vi "Update Wilt GUI.vi"(0 "Dryer In":T1 {"Night Cycle Count" format="%04d"; "Dryer Details"."Stop Dryer" items=["NO", "YES"]; "Dryer Details"."24 Hour Water Injection" items=["NO", "YES"]; "Dryer Details"."Run w/o Newfi" items=["NO", "YES"]; "Day Cycle Count" format="%04d"}, 1 "Day Shift?":bool, 2 "Enum":T5, 3 "Station Index":i32=13, 5 "Station Label In":string, 7 "New Dryer Details In":T2 {"Stop Dryer" items=["NO", "YES"]; "24 Hour Water Injection" items=["NO", "YES"]; "Run w/o Newfi" items=["NO", "YES"]}, 9 "Com Port In":u8=13, 11 "Dryer Status Serial Data In":T3, 12 "Agilent Data In":dbl[](array[numeric])=[1.0, 2.0, 3.0, 4.0, 5.0], 13 "Audit Alert":bool) -> (4 "Dryer Out 2":T1 {"Night Cycle Count" format="%04d"; "Dryer Details"."Stop Dryer" items=["NO", "YES"]; "Dryer Details"."24 Hour Water Injection" items=["NO", "YES"]; "Dryer Details"."Run w/o Newfi" items=["NO", "YES"]; "Day Cycle Count" format="%04d"}, 8 "New Dryer Testing File Init":bool, 10 "Restart Ready?":bool)   [LabVIEW 2012]
uses:
  Update Wilt GUI Control.ctl
  Dryer.ctl
  Dryer Details.ctl
  Dryer Com Port Info.ctl
  Dryer Status Ctrl.ctl
  Globals Wilt.vi
panel:
  in  "Tab Control":enum32{"Out", "In"}(tab)
  out "Dryer Breakout":T1 {"Night Cycle Count" format="%04d"; "Dryer Details"."Stop Dryer" items=["NO", "YES"]; "Dryer Details"."24 Hour Water Injection" items=["NO", "YES"]; "Dryer Details"."Run w/o Newfi" items=["NO", "YES"]; "Day Cycle Count" format="%04d"}
  in  "Dryer Out":T1 {"Night Cycle Count" format="%04d"; "Dryer Details"."Stop Dryer" items=["NO", "YES"]; "Dryer Details"."24 Hour Water Injection" items=["NO", "YES"]; "Dryer Details"."Run w/o Newfi" items=["NO", "YES"]; "Day Cycle Count" format="%04d"}
  out "Dryer Out.Sample Record(t, CC, Tc, ASCII, Status, L1,L2,Trmb,V{,V2,SW} )":string[](array[string])
  out "Dryer Out.Sample Record(t, CC, Tc, ASCII, Status, L1,L2,Trmb,V{,V2,SW} ) 2":string[](array[string])
  out "Dryer Breakout":T1 {"Night Cycle Count" format="%04d"; "Dryer Details"."Stop Dryer" items=["NO", "YES"]; "Dryer Details"."24 Hour Water Injection" items=["NO", "YES"]; "Dryer Details"."Run w/o Newfi" items=["NO", "YES"]; "Day Cycle Count" format="%04d"}
  in  "Dryer":T1 {"Night Cycle Count" format="%04d"; "Dryer Details"."Stop Dryer" items=["NO", "YES"]; "Dryer Details"."24 Hour Water Injection" items=["NO", "YES"]; "Dryer Details"."Run w/o Newfi" items=["NO", "YES"]; "Day Cycle Count" format="%04d"}
  # "D"
  # "N"
  # "D"
  # "N"
  # "D"
  # "N"
  # "D"
  # "N"
  # "D"
  # "N"
  # "D"
  # "N"
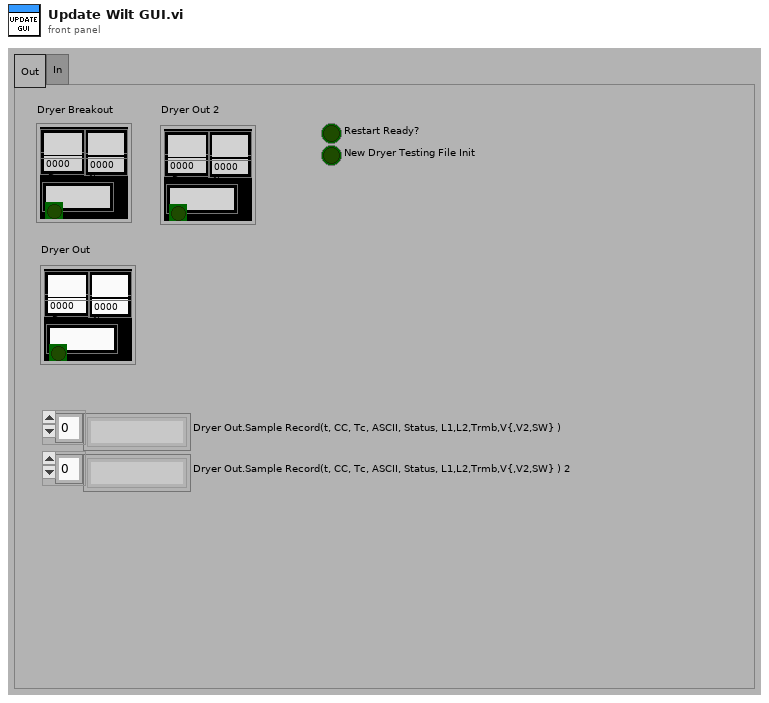
[diagram p1: front panel]
types:
  T1 = typedef "Dryer.ctl" = cluster{"Lab ID":string, "Day Cycle Count":i32, "Station Label":string, "Dryer Details":T2, "Sample Record ":string[], "Hist Record ":string[][], "Status Color":u32, "Boolean":bool, "Com Port":u8, "Bad Com Count":i32, "Current Run Start Time":dbl, "Night Cycle Count":i32, "Station Index":i32, "Cycle Index":string, "Audit Alert":bool}
  T2 = typedef "Dryer Details.ctl" = cluster{"Station":string, "Cycle Count Day":string, "Status":string, "Debug ASCII":string, "Notes":string, "Lab ID":string, "Total Time On":string, "TR Number":string, "Cycle Count Night":string, "Time On Day":string, "Time On Night":string, "Run w/o Newfi":i32, "24 Hour Water Injection":i32, "Stop Dryer":i32}
  T3 = typedef "Dryer Com Port Info.ctl" = cluster{"Color":u32, "Last Read Status":T4, "Command:Data":string, "Com Port":u8, "Time(S)":dbl, "Err Count":u32}
  T4 = typedef "Dryer Status Ctrl.ctl" = enum16{"Cycle Not Started", "Cycle Running", "Paused", "Cycle Completed", "Eval Mode Entered", "Err", "Pause (No GEA2)"}
  T5 = typedef "Update Wilt GUI Control.ctl" = enum16{"Init Station Number", "Update Detail Data", "Update Status", "Init Com Port Num", "Update Sample Info", "Reset All Cycles"}
  T6 = cluster{"New Dryer Details In":T2, "Station Label In":string, "Com Port In":u8, "Agilent Data In":dbl[], "Dryer Status Serial Data In":T3, "Restart Ready?":bool, "Dryer Out":T1, "Temperature Fault":bool, "Station Index":i32, "Audit Alert":bool, "Day Shift?":bool}
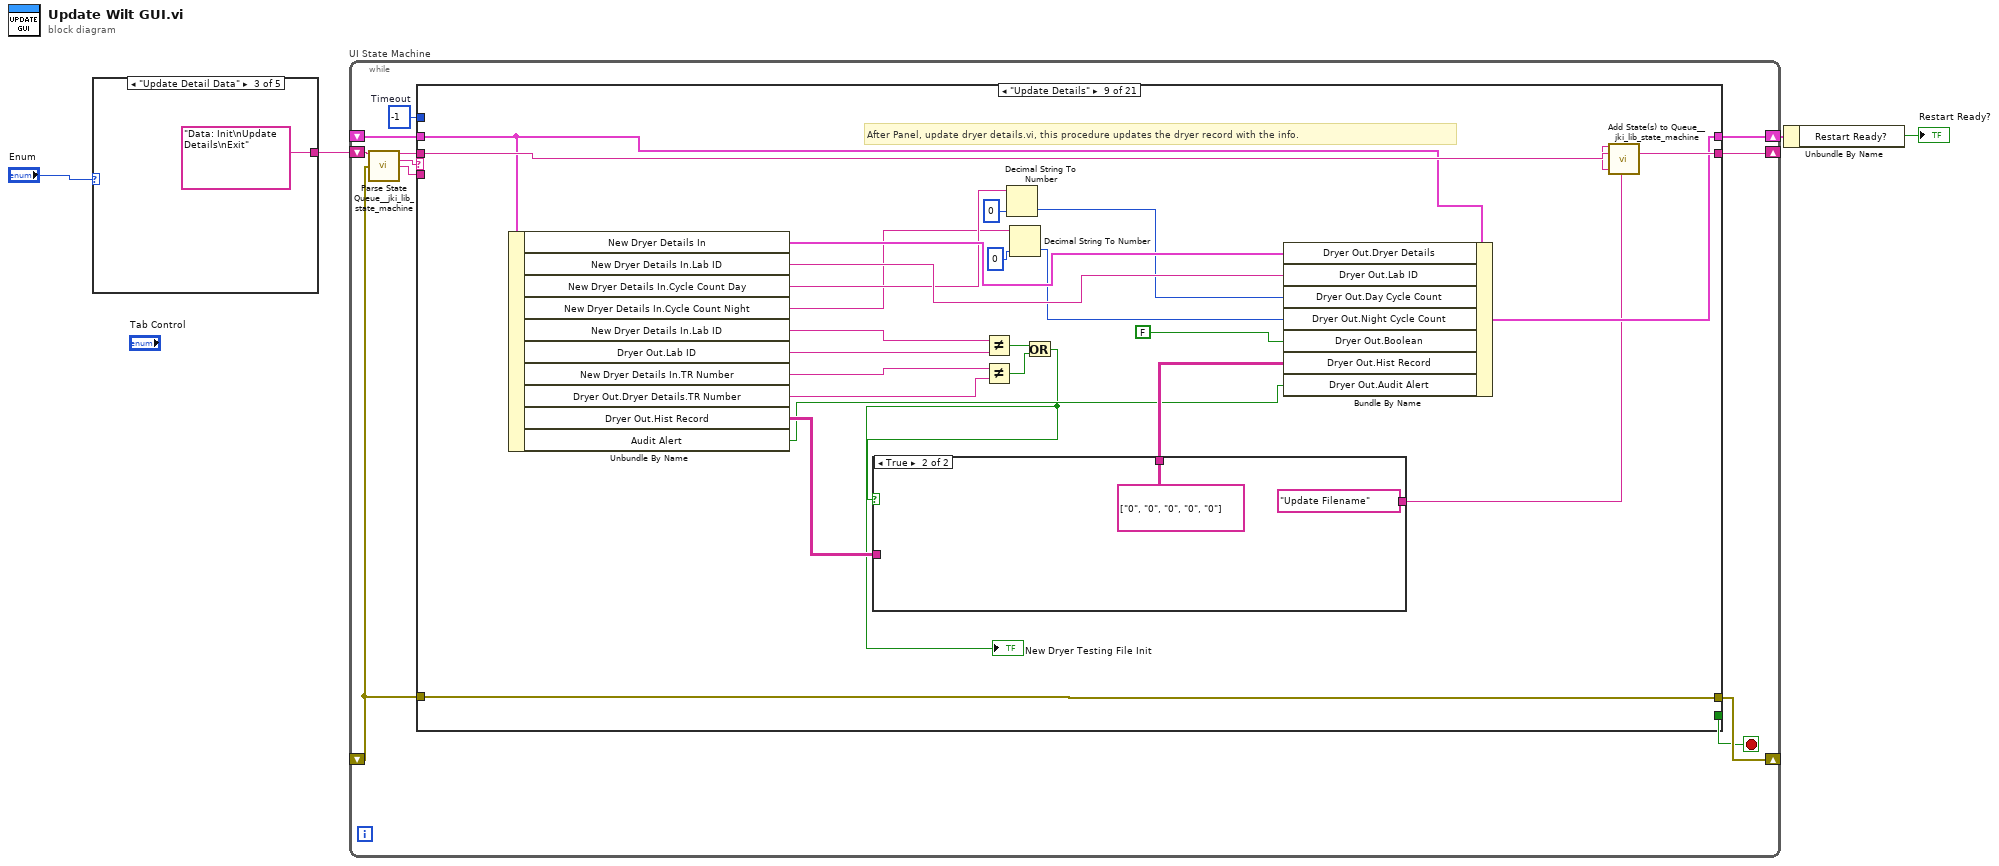
[diagram p0: block diagram]
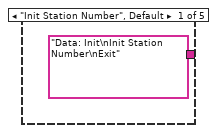
[diagram p2: hidden frame]
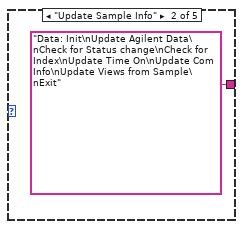
[diagram p3: hidden frame]
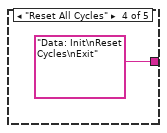
[diagram p4: hidden frame]
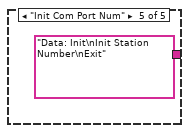
[diagram p5: hidden frame]
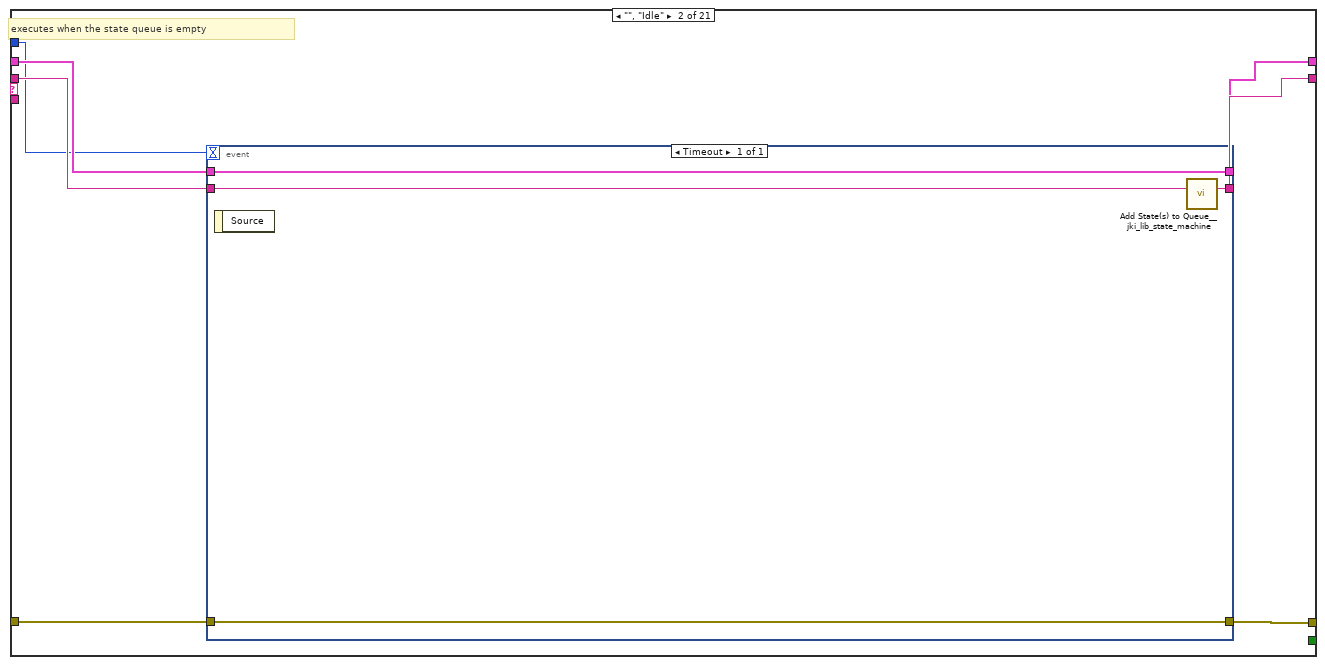
[diagram p7: hidden frame]
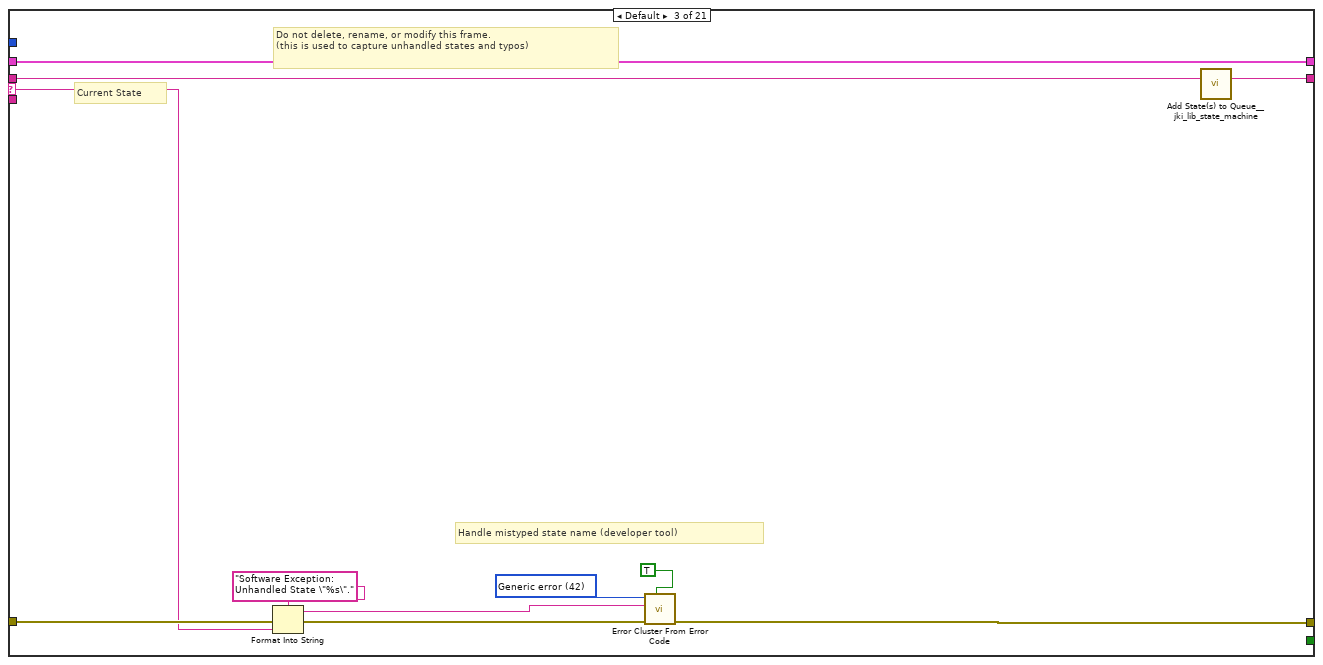
[diagram p8: hidden frame]
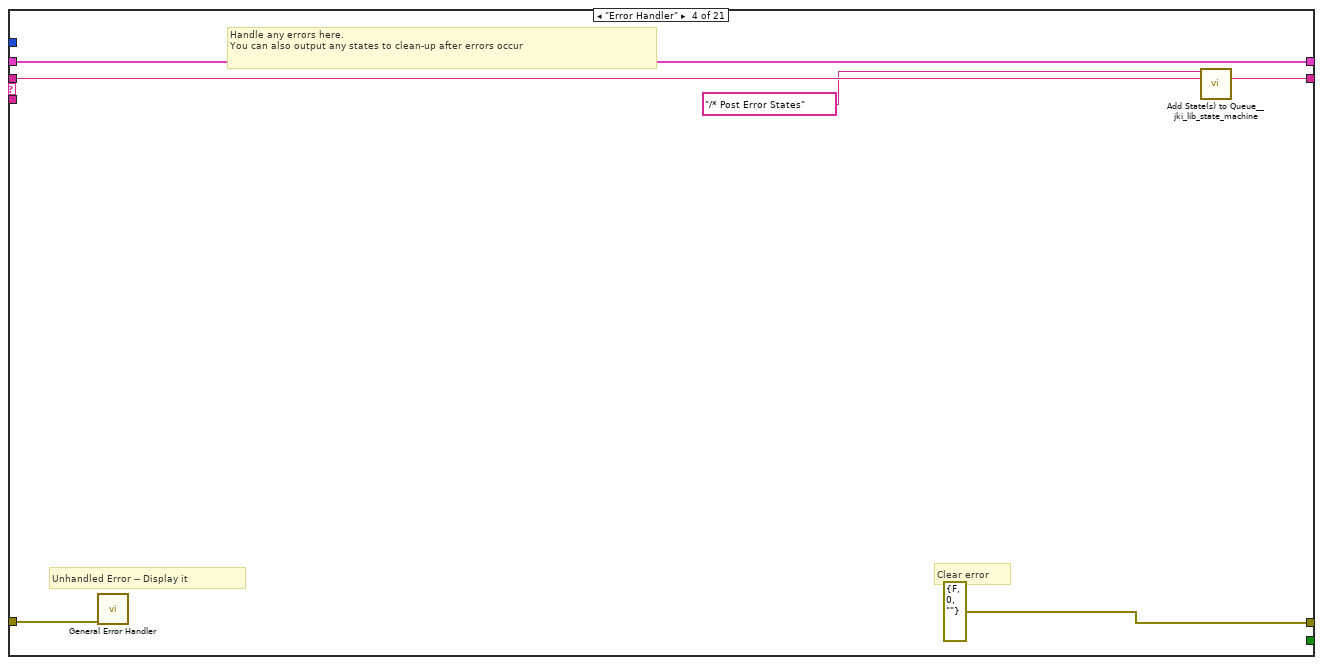
[diagram p9: hidden frame]
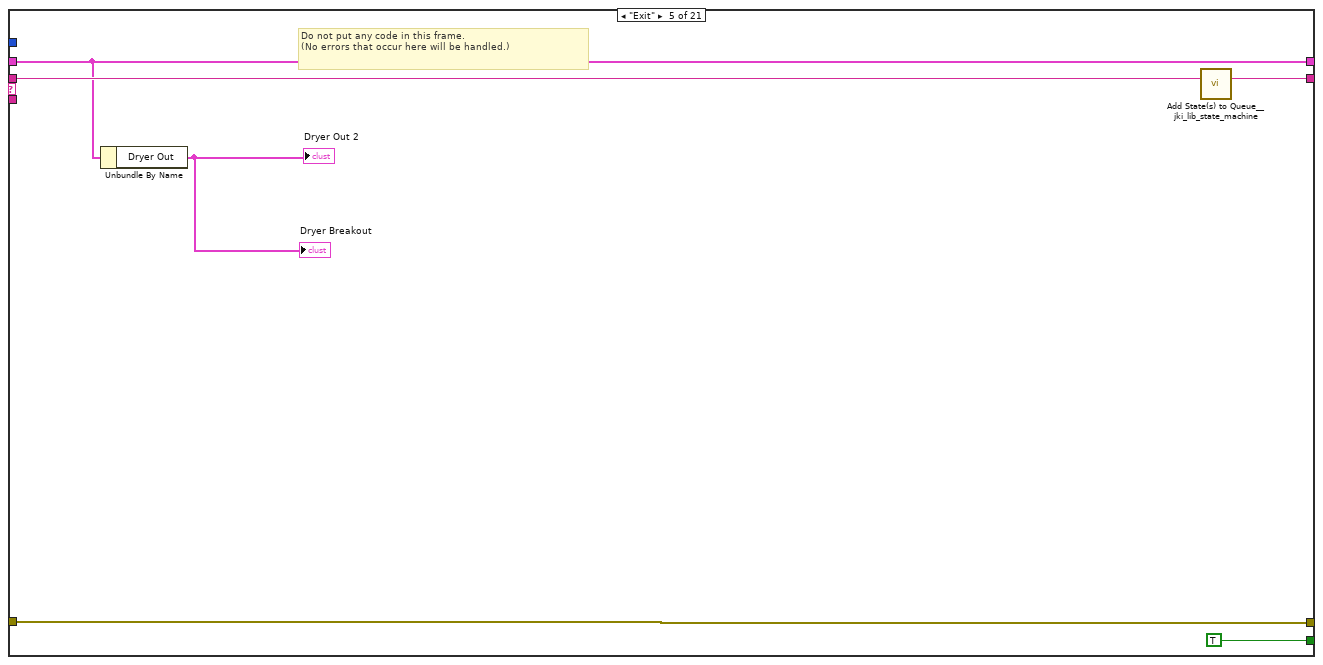
[diagram p10: hidden frame]
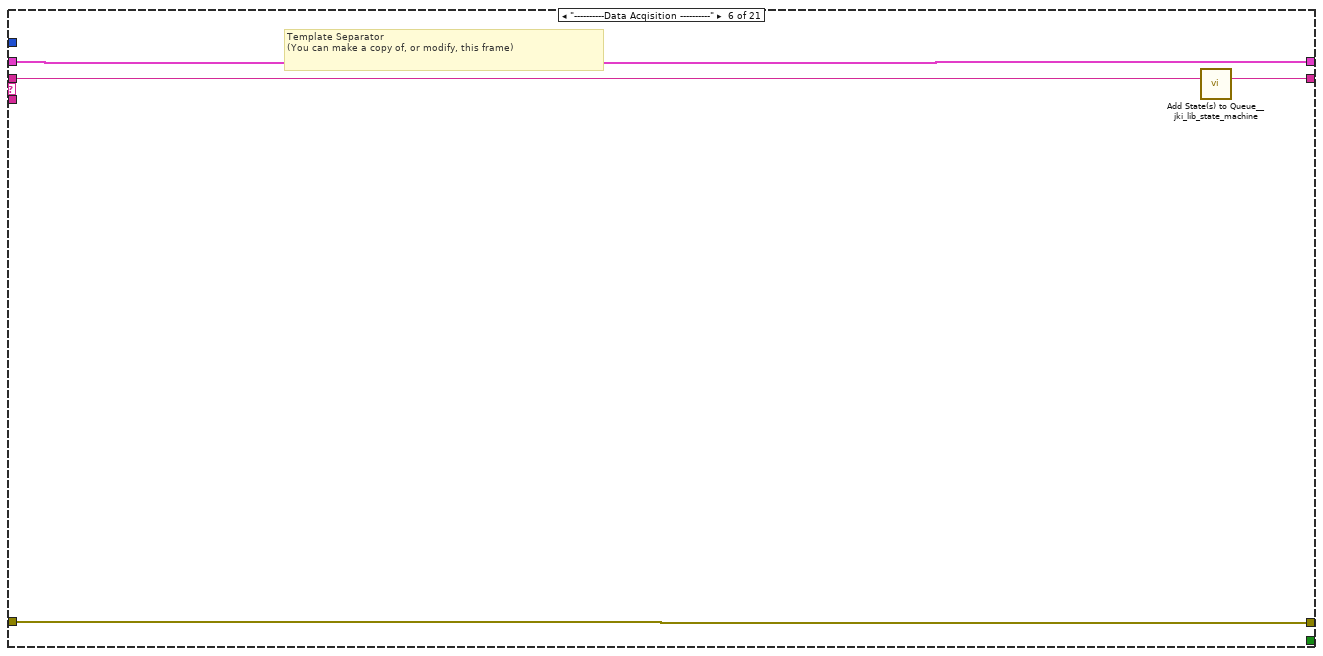
[diagram p11: hidden frame]
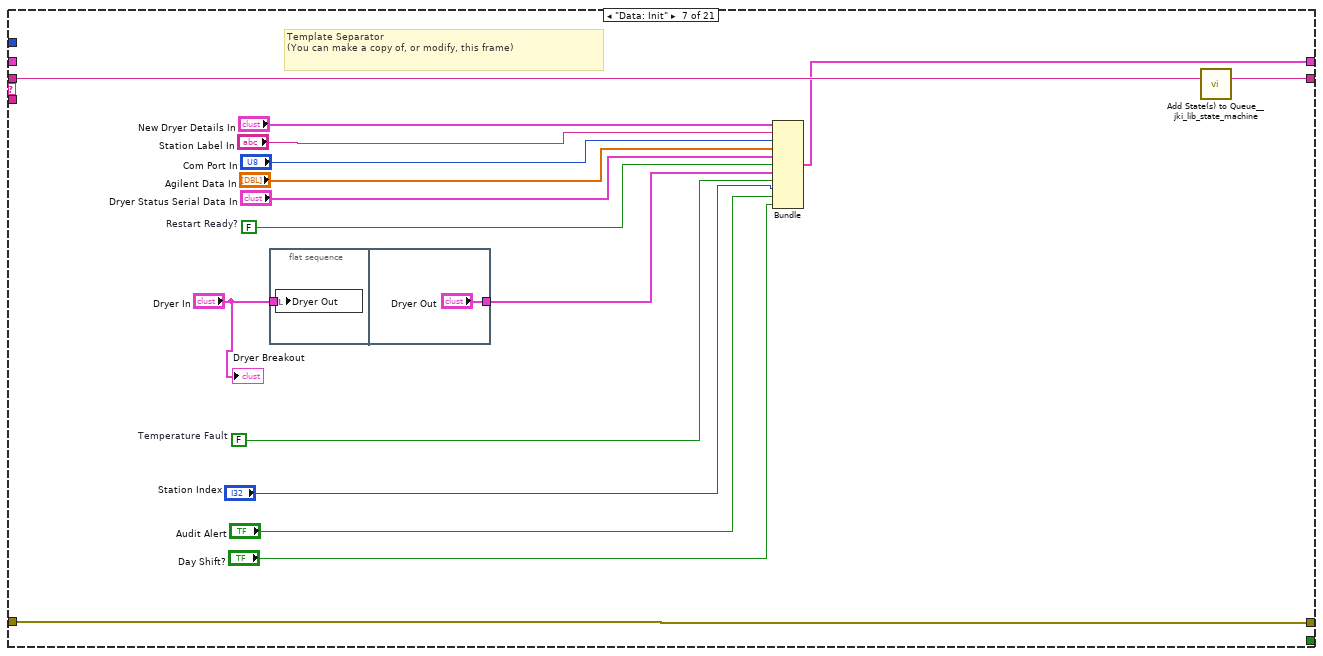
[diagram p12: hidden frame]
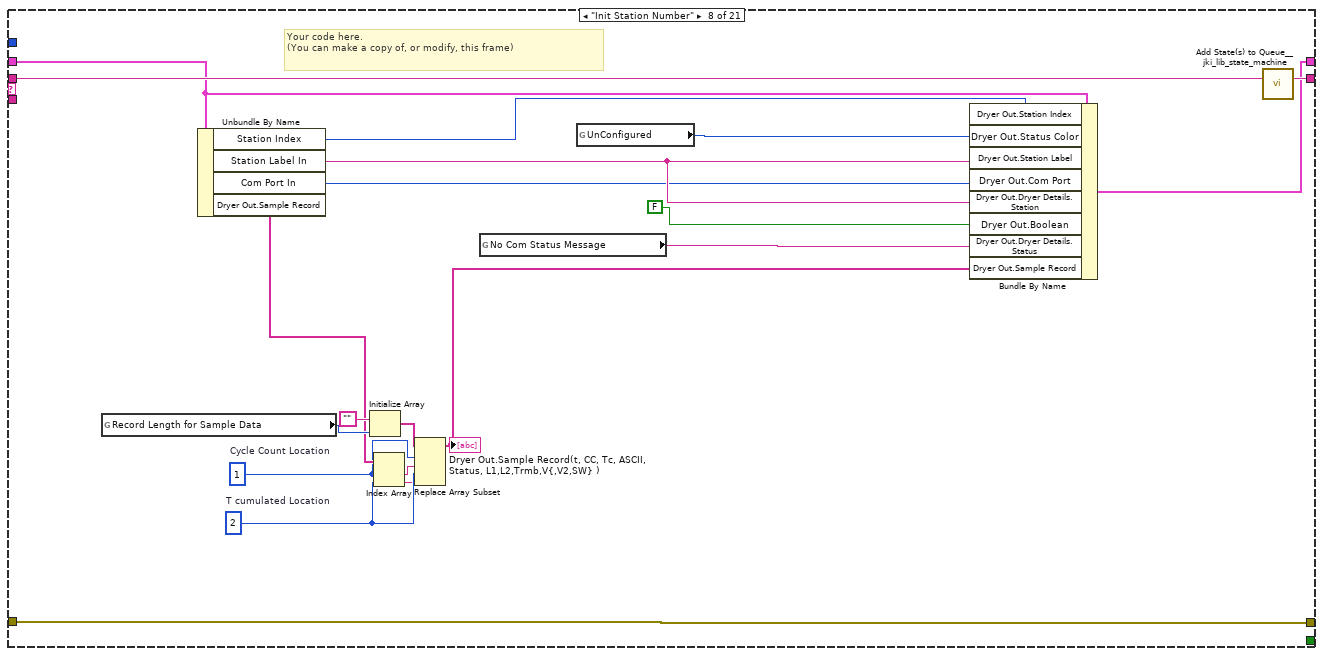
[diagram p13: hidden frame]
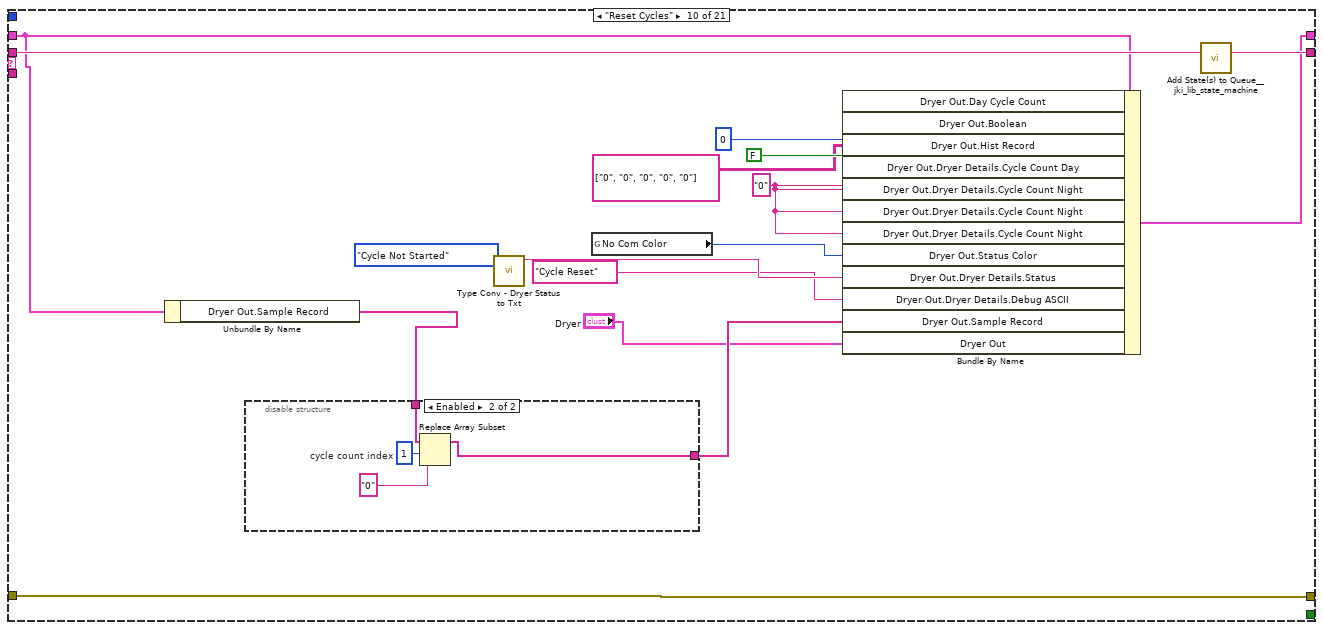
[diagram p15: hidden frame]
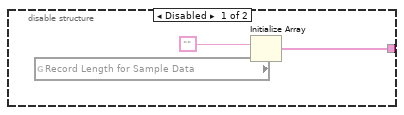
[diagram p16: hidden frame]
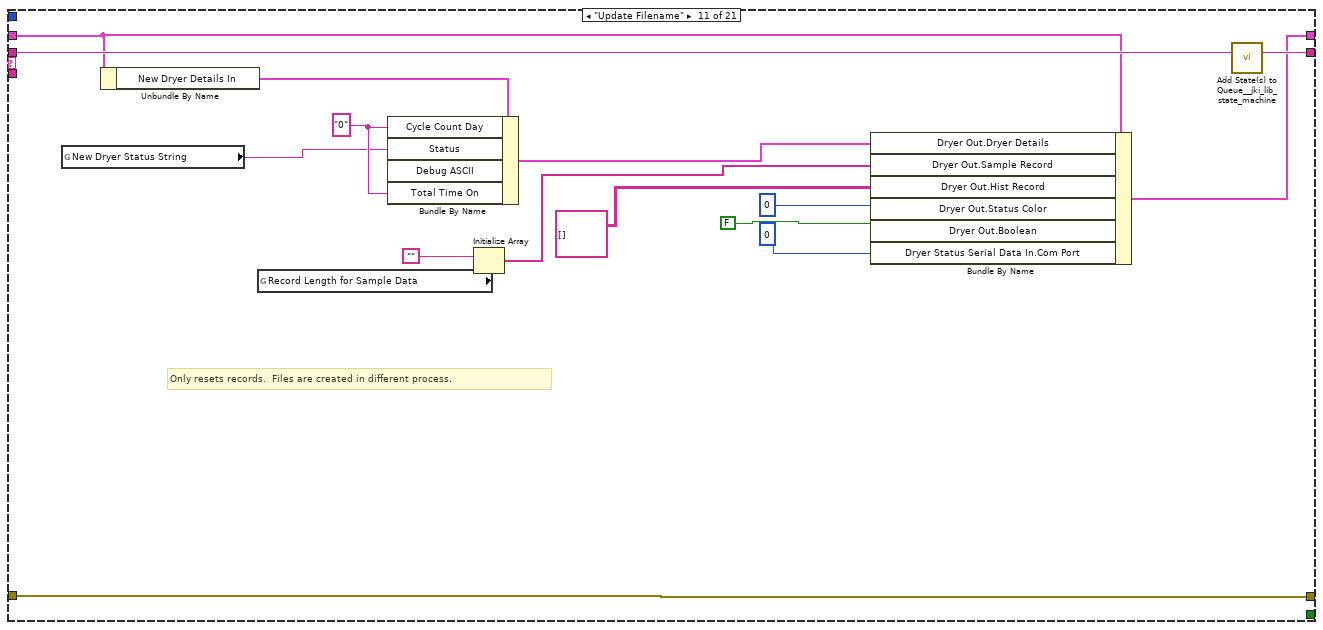
[diagram p17: hidden frame]
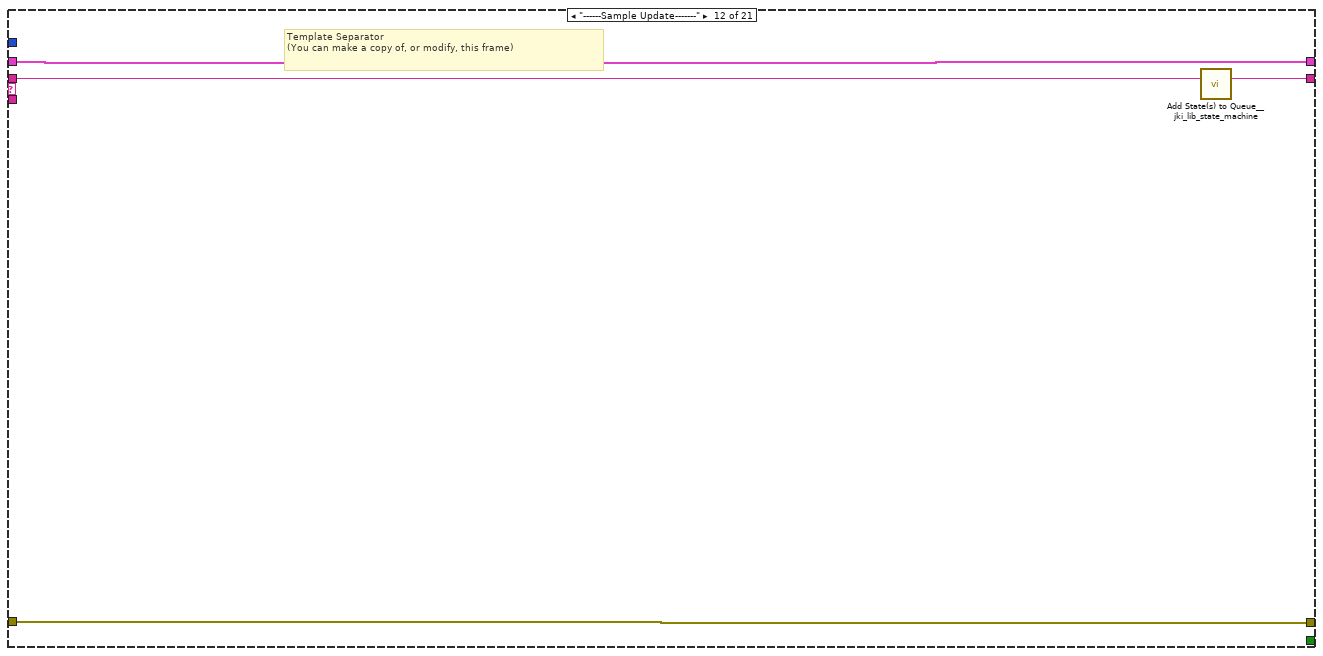
[diagram p18: hidden frame]
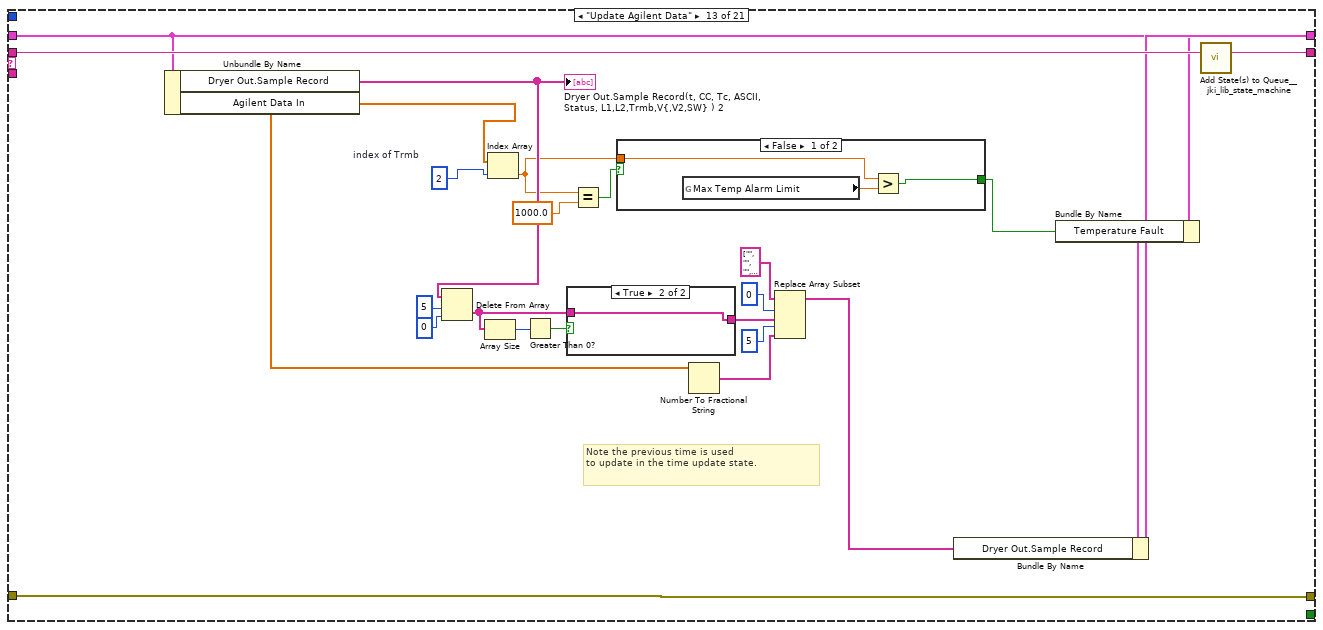
[diagram p19: hidden frame]
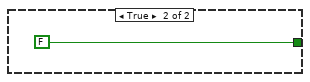
[diagram p20: hidden frame]
diagram:
  n1 = case shown="\"Update Detail Data\"" "Enum" {
    tunnel: ["Data: Init\nInit Station Number\nExit" ("States Out") "Data: Init\nUpdate Agilent Data\nCheck for Status change\nCheck for Index\nUpdate Time On\nUpdate Com Info\nUpdate Views from Sample\nExit" ("States Out") "Data: Init\nUpdate Details\nExit" ("States Out") "Data: Init\nReset Cycles\nExit" ("States Out") "Data: Init\nInit Station Number\nExit" ("States Out")] -> w3
    frame "Init Station Number", Default {
    }
    frame "Update Sample Info" {
    }
    frame "Update Detail Data" {
    }
    frame "Reset All Cycles" {
    }
    frame "Init Com Port Num" {
    }
  }
  n2 = while "UI State Machine" {
    shift-right: [w13] -> w2
    shift-left: _ -> [w12]
    shift-right: [w16] -> _
    shift-left: _ -> [w10]
    shift-right: [w15] -> _
    shift-left: w3 -> [w17]
    stop <- w14 stop-if-true
    w11 = -1  # Timeout
    n3 = call <vilib>:"Parse State Queue__jki_lib_state_machine.vi"("State Queue"=w17, "Error In (no error)"=w10) -> ("Remaining States"=w19:string, "Current State"=w20:string, "Arguments"=w18:string)  [unwired: 11 in]
    n4 = case shown="\"Update Details\"" w20 {
      selector: w20 -> [_ _ w35 _ _ _ _ _ _ _ _ _ _ _ _ _ _ _ _ _ _]
      tunnel: w19 -> [w22 w30 w39 w51 w57 w61 w77 w99 w124 w143 w166 w170 w194 w215 w263 w294 w363 w417 w421 w440 w464]
      tunnel: w18 -> [_ _ _ _ _ _ _ _ _ _ _ _ _ _ _ _ _ _ _ _ _]
      tunnel: w12 -> [w23 w28 w37 w48 w53 w58 _ w80 w117 w131 w163 w167 w187 w207 w259 w288 w360 w414 w418 w437 w460]
      tunnel: [w21 w27 w41 errorcluster {"status"=FALSE, "code"=0, "source"=""} ("error out") w55 w59 w75 w97 w122 w141 w164 w168 w192 w213 w261 w292 w361 w415 w419 w438 w462] -> w16
      tunnel: w10 -> [w21 w26 w40 w47 w55 w59 w75 w97 w122 w141 w164 w168 w192 w213 w261 w292 w361 w415 w419 w438 w462]
      tunnel: [w22 w29 w38 w50 w56 w60 w76 w98 w123 w142 w165 w169 w193 w214 w262 w293 w362 w416 w420 w439 w463] -> w15
      tunnel: [_ _ _ _ TRUE _ _ _ _ _ _ _ _ _ _ _ _ _ _ _ _] -> w14
      tunnel: [w23 w25 w37 w48 w53 w58 w74 w96 w121 w140 w162 w167 w191 w206 w258 w287 w359 w413 w418 w436 w459] -> w13
      tunnel: w11 -> [_ w24 _ _ _ _ _ _ _ _ _ _ _ _ _ _ _ _ _ _ _]
      frame "ABOUT" {
        # "TAKES DATA FROM DRYER COM INFO AND INTEGRATES IT INTO THE RECORD."
        # "Update Dryer WILT data structure\nwith new data, or init:"
      }
      frame "", "Idle" {
        # "executes when the state queue is empty"
        n5 = event shown="[0] Timeout" {
          selector: _ -> [_]
          dyn-events: _ -> [_]
          timeout: w24 -> [_]
          tunnel: w30 -> [w34]
          tunnel: [w33] -> w29
          tunnel: w28 -> [w31]
          tunnel: [w32] -> w27
          tunnel: w26 -> [w32]
          tunnel: [w31] -> w25
          event Timeout {
            n6 = event-data() -> ()  [unwired: 1 in, 1 out]
            n7 = call <vilib>:"Add State(s) to Queue__jki_lib_state_machine.vi"("State(s) in (\"\")"=w34) -> ("States Out"=w33:string)  [unwired: 14 in]
          }
        }
      }
      frame Default {
        w44 = 42 items=["No error", "Argument error", "Memory is full", "Out of zone", "End of file", "File already open", "Generic file I/O error", "File not found", "File permission error", "Disk is full", "Duplicate path", "Too many files open", "System feature not enabled", "Resource file not found", "Cannot add resource", "Resource not found", "Image not found", "Image memory error", "Pen does not exist", "Config type invalid", "Config token not found", "Config parse error", "Config memory error", "Bad external code format", "Bad external code offset", "External code not present", "Null window", "Destroy window error", "Null menu", "Print aborted", "Bad print record", "Print driver error", "Windows error during printing", "Memory error during printing", "Print dialog error", "Generic print error", "Invalid device refnum", "Device not found", "Device parameter error", "Device unit error", "Cannot open device", "Device call aborted", "Generic error", "Cancelled by user", "Object ID too low", "Object ID too high", "Object not in heap", "Unknown heap", "Unknown object (invalid DefProc)", "Unknown object (DefProc not in table)", "Message out of range", "Invalid (null) method", "Unknown message", "Manager call not supported", "Bad address", "Network operation in progress", "Network operation timed out", "Connection is busy", "Network attribute not supported", "Network error", "Address in use", "System out of memory", "Connection aborted", "Connection refused", "Not connected", "Already connected", "Connection closed", "Initialization error (interapplication manager)", "Bad occurrence", "Wait on unbound occurrence handler", "Occurrence queue overflow", "Datalog type conflict", "Unused", "Unrecognized type (interapplication manager)", "Memory corrupt", "Failed to make temporary DLL", "Old CIN version", "Drag socket not found", "Failed to load drop-object", "Failed to register OLE object", "Failed to release OLE object", "Format specifier type mismatch", "Unknown format specifier", "Too few format specifiers", "Too many format specifiers", "Scan failed", "Newer CIN version", "Error converting to variant", "Runtime menu error", "Password tampered", "Variant attribute not found", "Incompatible variant data type", "Event data is not available", "Event Store is not present", "Occurrence is not found", "Event Queue is not created", "Event info is not available", "Refnum passed is NULL", "Error retrieving Class GUID", "Error retrieving CoClass GUID", "Error retrieving TypeLib GUID.", "Bad built application magic bytes.", "Specific driver is different from the specific driver associated with the Logical Name.", "There is no session opened to the class driver.", "Max Error", "MAX - Error with config objects", "MAX - Error loading configuration", "MAX - Group not supported"]
        # "Current State"
        # "Do not delete, rename, or modify this frame.\n(this is used to capture unhandled states and typos)"
        # "Handle mistyped state name (developer tool)"
        n8 = Format Into String(format string="Software Exception: Unhandled State \"%s\"." ("message"), error in=w40, w35) -> (resulting string=w43:string, error out=w42:errorcluster)  [unwired: 1 in]
        n9 = call <vilib>:"Error Cluster From Error Code.vi"("show call chain? (False)"=TRUE, "error in (no error)"=w42, "error message (\"\")"=w43, "error code (0)"=w44) -> ("error out"=w41:errorcluster)  [unwired: 5 in]
        n10 = call <vilib>:"Add State(s) to Queue__jki_lib_state_machine.vi"("State(s) in (\"\")"=w39) -> ("States Out"=w38:string)  [unwired: 14 in]
      }
      frame "Error Handler" {
        # "Unhandled Error -- Display it"
        # "Handle any errors here.\nYou can also output any states to clean-up after errors occur"
        # "Clear error"
        n11 = call <vilib>:"General Error Handler.vi"("error in (no error)"=w47) -> ()  [unwired: 10 in, 5 out]
        n12 = call <vilib>:"Add State(s) to Queue__jki_lib_state_machine.vi"("State(s) in Front (\"\")"="/* Post Error States", "State(s) in (\"\")"=w51) -> ("States Out"=w50:string)  [unwired: 13 in]
      }
      frame "Exit" {
        # "Do not put any code in this frame.\n(No errors that occur here will be handled.)"
        n13 = Unbundle By Name(w53) -> ("Dryer Out"=→"Dryer Out 2" →"Dryer Breakout":T1)
        n14 = call <vilib>:"Add State(s) to Queue__jki_lib_state_machine.vi"("State(s) in (\"\")"=w57) -> ("States Out"=w56:string)  [unwired: 14 in]
      }
      frame "----------Data Acqisition ----------" {
        # "Template Separator\n(You can make a copy of, or modify, this frame)"
        n15 = call <vilib>:"Add State(s) to Queue__jki_lib_state_machine.vi"("State(s) in (\"\")"=w61) -> ("States Out"=w60:string)  [unwired: 14 in]
      }
      frame "Data: Init" {
        w66 = FALSE  # Temperature Fault
        w69 = FALSE  # Restart Ready?
        # "Template Separator\n(You can make a copy of, or modify, this frame)"
        n16 = flat-sequence {
          tunnel: "Dryer In" -> [w78]
          tunnel: ["Dryer Out"] -> w67
          frame #0 {
            n17 = local write "Dryer Out"(w78) -> ()
          }
          frame #1 {
          }
        }
        n18 = Bundle("New Dryer Details In"="New Dryer Details In", "Station Label In"="Station Label In", "Com Port In"="Com Port In", "Agilent Data In"="Agilent Data In", "Dryer Status Serial Data In"="Dryer Status Serial Data In", "Restart Ready?"=w69, "Dryer Out"=w67, "Temperature Fault"=w66, "Station Index"="Station Index", "Audit Alert"="Audit Alert", "Day Shift?"="Day Shift?") -> (w74:T6)  [unwired: 1 in]
        n19 = call <vilib>:"Add State(s) to Queue__jki_lib_state_machine.vi"("State(s) in (\"\")"=w77) -> ("States Out"=w76:string)  [unwired: 14 in]
        "Dryer Breakout" <- "Dryer In"
      }
      frame "Init Station Number" {
        w85 = 2  # T cumulated Location
        w87 = 1  # Cycle Count Location
        # "Your code here.\n(You can make a copy of, or modify, this frame)"
        n20 = global read "Globals Wilt.vi" "Record Length for Sample Data"() -> (w91:i32)
        n21 = Unbundle By Name(w80) -> ("Station Index"=w81:i32, "Station Label In"=w83:string, "Com Port In"=w82:u8, "Dryer Out.Sample Record"=w88:string[])
        n22 = Initialize Array("", w91) -> (w90:string[])
        n23 = Index Array(array=w88, index #1=w87, index #2=w85) -> (element #1=w86:string, element #2=w84:string)
        n24 = Replace Array Subset(array=w90, new element #1=w86, index #1=w87, new element #2=w84, index #2=w85) -> (w89:string[])
        "Dryer Out.Sample Record(t, CC, Tc, ASCII, Status, L1,L2,Trmb,V{,V2,SW} )" <- w89
        n25 = global read "Globals Wilt.vi" "No Com Status Message"() -> (w93:string)
        n26 = global read "Globals Wilt.vi" "UnConfigured"() -> (w94:u32)
        n27 = Bundle By Name(cluster=w80, "Dryer Out.Station Index"=w81, "Dryer Out.Status Color"=w94, "Dryer Out.Station Label"=w83, "Dryer Out.Com Port"=w82, "Dryer Out.Dryer Details.Station"=w83, "Dryer Out.Boolean"=FALSE ("Dryer In.Boolean"), "Dryer Out.Dryer Details.Status"=w93, "Dryer Out.Sample Record"=w89) -> (w96:T6)
        n28 = call <vilib>:"Add State(s) to Queue__jki_lib_state_machine.vi"("State(s) in (\"\")"=w99) -> ("States Out"=w98:string)  [unwired: 14 in]
      }
      frame "Update Details" {
        # "After Panel, update dryer details.vi, this procedure updates the dryer record with the info."
        n29 = Unbundle By Name(w117) -> ("New Dryer Details In"=w111:T2, "New Dryer Details In.Lab ID"=w109:string, "New Dryer Details In.Cycle Count Day"=w108:string, "New Dryer Details In.Cycle Count Night"=w105:string, "New Dryer Details In.Lab ID"=w103:string, "Dryer Out.Lab ID"=w102:string, "New Dryer Details In.TR Number"=w104:string, "Dryer Out.Dryer Details.TR Number"=w116:string, "Dryer Out.Hist Record"=w112:string[][], "Audit Alert"=w101:bool)
        n30 = Not Equal?(x=w103, y=w102) -> (x != y?=w115:bool)
        n31 = Not Equal?(x=w104, y=w116) -> (x != y?=w114:bool)
        n32 = Decimal String To Number(string=w108, default (0L)=0 ("default (0 I32)")) -> (number=w107:i32)  [unwired: 1 in, 1 out]
        n33 = Decimal String To Number(string=w105, default (0L)=0 ("default (0 I32)")) -> (number=w106:i32)  [unwired: 1 in, 1 out]
        n34 = Or(x=w115, y=w114) -> (x .or. y?=w100:bool)
        "New Dryer Testing File Init" <- w100
        n35 = case shown="True" w100 {
          tunnel: [_ "Update Filename"] -> w120
          tunnel: [w125 string[][] [["0", "0", "0", "0", "0"]] ("Hist Record(Cycle Count, t-comp,L1max, L2max, Tmax)")] -> w113
          tunnel: w112 -> [w125 _]
          frame False {
          }
          frame True {
          }
        }
        n36 = Bundle By Name(cluster=w117, "Dryer Out.Dryer Details"=w111, "Dryer Out.Lab ID"=w109, "Dryer Out.Day Cycle Count"=w107, "Dryer Out.Night Cycle Count"=w106, "Dryer Out.Boolean"=FALSE ("Dryer In.Boolean"), "Dryer Out.Hist Record"=w113, "Dryer Out.Audit Alert"=w101) -> (w121:T6)
        n37 = call <vilib>:"Add State(s) to Queue__jki_lib_state_machine.vi"("State(s) in Front (\"\")"=w120, "State(s) in (\"\")"=w124) -> ("States Out"=w123:string)  [unwired: 13 in]
      }
      frame "Reset Cycles" {
        w128 = "0" ("Dryer Out.Dryer Details.Cycle Count")
        n38 = Unbundle By Name(w131) -> ("Dryer Out.Sample Record"=w130:string[])
        n39 = disable-structure shown="Enabled" {
          disable-tunnel: [w144 w147] -> w132
          disable-tunnel: w130 -> [_ w150]
          frame Disabled {
            n40 = global read "Globals Wilt.vi" "Record Length for Sample Data"() -> (w145:i32)
            n41 = Initialize Array("", w145) -> (w144:string[])
          }
          frame Enabled {
            w149 = 1  # cycle count index
            n42 = Replace Array Subset(array=w150, new element="0" ("new element/subarray"), index=w149) -> (w147:string[])
          }
        }
        n43 = call "Type Conv - Dryer Status to Txt.vi"("Status"=Dryer_Status_Ctrl."Cycle Not Started") -> ("Ring Text.Text"=w134:string)  [unwired: 10 in]
        n44 = global read "Globals Wilt.vi" "No Com Color"() -> (w136:u32)
        n45 = Bundle By Name(cluster=w131, "Dryer Out.Day Cycle Count"=0 ("Dryer Out.Cycle Count"), "Dryer Out.Boolean"=FALSE ("Dryer In.Boolean"), "Dryer Out.Hist Record"=string[][] [["0", "0", "0", "0", "0"]] ("Hist Record(Cycle Count, t-comp,L1max, L2max, Tmax)"), "Dryer Out.Dryer Details.Cycle Count Day"=w128, "Dryer Out.Dryer Details.Cycle Count Night"=w128, "Dryer Out.Dryer Details.Cycle Count Night"=w128, "Dryer Out.Dryer Details.Cycle Count Night"=w128, "Dryer Out.Status Color"=w136, "Dryer Out.Dryer Details.Status"=w134, "Dryer Out.Dryer Details.Debug ASCII"="Cycle Reset", "Dryer Out.Sample Record"=w132, "Dryer Out"="Dryer") -> (w140:T6)
        n46 = call <vilib>:"Add State(s) to Queue__jki_lib_state_machine.vi"("State(s) in (\"\")"=w143) -> ("States Out"=w142:string)  [unwired: 14 in]
      }
      frame "Update Filename" {
        w161 = "0" ("Cycle Count")
        # "Only resets records.  Files are created in different process."
        n47 = global read "Globals Wilt.vi" "New Dryer Status String"() -> (w151:string)
        n48 = Unbundle By Name(w163) -> ("New Dryer Details In"=w159:T2)
        n49 = global read "Globals Wilt.vi" "Record Length for Sample Data"() -> (w152:i32)
        n50 = Bundle By Name(cluster=w159, "Cycle Count Day"=w161, "Status"=w151, "Debug ASCII"=w151, "Total Time On"=w161) -> (w160:T2)
        n51 = Initialize Array("", w152) -> (w153:string[])
        n52 = Bundle By Name(cluster=w163, "Dryer Out.Dryer Details"=w160, "Dryer Out.Sample Record"=w153, "Dryer Out.Hist Record"=string[][] [] ("Dryer In.Sample Record(t, CC, Tc, ASCII, Status, L1,L2,Trmb,V{,V2,SW} )"), "Dryer Out.Status Color"=u32 0 ("Dryer In.Status Color"), "Dryer Out.Boolean"=FALSE ("Dryer In.Boolean"), "Dryer Status Serial Data In.Com Port"=u8 0 ("Dryer In.Com Port")) -> (w162:T6)
        n53 = call <vilib>:"Add State(s) to Queue__jki_lib_state_machine.vi"("State(s) in (\"\")"=w166) -> ("States Out"=w165:string)  [unwired: 14 in]
      }
      frame "------Sample Update-------" {
        # "Template Separator\n(You can make a copy of, or modify, this frame)"
        n54 = call <vilib>:"Add State(s) to Queue__jki_lib_state_machine.vi"("State(s) in (\"\")"=w170) -> ("States Out"=w169:string)  [unwired: 14 in]
      }
      frame "Update Agilent Data" {
        w175 = 2  # index of Trmb
        # "Note the previous time is used\nto update in the time update state."
        n55 = Unbundle By Name(w187) -> ("Dryer Out.Sample Record"=w188:string[], "Agilent Data In"=w190:dbl[])
        "Dryer Out.Sample Record(t, CC, Tc, ASCII, Status, L1,L2,Trmb,V{,V2,SW} ) 2" <- w188
        n56 = Delete From Array(array=w188, length=5, index=0) -> (deleted portion=w181:string[])  [unwired: 1 out]
        n57 = Array Size(array=w181) -> (size(s)=w183:i32)
        n58 = Index Array(array=w190, index=w175) -> (element=w171:dbl)
        n59 = Greater Than 0?(x=w183) -> (x > 0?=w182:bool)
        n60 = case shown="True" w182 {
          tunnel: [string[] ["0", "0", "0", "ASCII", " STAT"] w200] -> w178
          tunnel: w181 -> [_ w200]
          frame False {
          }
          frame True {
          }
        }
        n61 = Equal?(x=w171, y=1000.0) -> (x = y?=w173:bool)
        n62 = case shown="False" w173 {
          tunnel: [w195 FALSE] -> w172
          tunnel: w171 -> [w196 _]
          frame False {
            n63 = global read "Globals Wilt.vi" "Max Temp Alarm Limit"() -> (w197:dbl)
            n64 = Greater?(x=w196, y=w197) -> (0:w195:bool)
          }
          frame True {
          }
        }
        n65 = Number To Fractional String(number=w190) -> (F-format string=w176:string[])  [unwired: 3 in]
        n66 = Replace Array Subset(array=string[] ["", "", "", "", "", "", "", "", "", "", " "], new element #1=w178, index #1=0 ("index"), new element #2=w176, index #2=5 ("index")) -> (w189:string[])
        n67 = Bundle By Name(cluster=w187, "Temperature Fault"=w172) -> (w186:T6)
        n68 = Bundle By Name(cluster=w186, "Dryer Out.Sample Record"=w189) -> (w191:T6)
        n69 = call <vilib>:"Add State(s) to Queue__jki_lib_state_machine.vi"("State(s) in (\"\")"=w194) -> ("States Out"=w193:string)  [unwired: 14 in]
      }
      frame "Check for Status change" {
        w203 = 4  # Status Location
        # "new stat"
        # "old stat"
        # "If the status string changes from:\n1. running to complete: set restart ready\n2. complete to running: go to increment count."
        n70 = Unbundle By Name(w207) -> ("Dryer Out.Hist Record"=w202:string[][], "Dryer Out.Current Run Start Time"=w201:dbl, "Dryer Out.Sample Record"=w211:string[], "Dryer Status Serial Data In"=w212:T3)
        n71 = Unbundle By Name(w212) -> ("Last Read Status"=w210:T4)
        n72 = call "Type Conv - Dryer Status to Txt.vi"("Status"=w210) -> ("Ring Text.Text"=w204:string)  [unwired: 10 in]
        n73 = Index Array(array=w211, index=w203) -> (element=w205:string)
        n74 = Equal?(x=w205, y=w204) -> (x = y?=w209:bool)
        n75 = case shown="False" w209 {
          tunnel: [w228 "" ("State(s) in Front (\"\")")] -> w208
          tunnel: w204 -> [w235 _]
          tunnel: w205 -> [w234 _]
          tunnel: w207 -> [w225 w250]
          tunnel: [w224 w250] -> w206
          tunnel: w202 -> [w221 _]
          tunnel: w201 -> [w219 _]
          frame False {
            # "end"
            # "start"
            # "new stat"
            # "old stat"
            n76 = call "E-Time.vi"() -> ("Elapsed Time (sec)"=w220:dbl)  [unwired: 9 in, 2 out]
            n77 = call "Type Conv - Dryer Status to Txt.vi"("Status"=Dryer_Status_Ctrl."Cycle Completed") -> ("Ring Text.Text"=w232:string)  [unwired: 10 in]
            n78 = call "Type Conv - Dryer Status to Txt.vi"("Status"=Dryer_Status_Ctrl."Cycle Running") -> ("Ring Text.Text"=w233:string)  [unwired: 10 in]
            n79 = call "Type Conv - Dryer Status to Txt.vi"("Status"=Dryer_Status_Ctrl."Cycle Running") -> ("Ring Text.Text"=w237:string)  [unwired: 10 in]
            n80 = call "Type Conv - Dryer Status to Txt.vi"("Status"=Dryer_Status_Ctrl."Cycle Completed") -> ("Ring Text.Text"=w236:string)  [unwired: 10 in]
            n81 = Subtract(x=w220, y=w219) -> (x-y=w218:dbl)
            n82 = Concatenate Strings(w235, w234) -> (w226:string)
            n83 = Concatenate Strings(w232, w233) -> (w229:string)
            n84 = Concatenate Strings(w237, w236) -> (w227:string)
            n85 = Number To Fractional String(number=w218, precision (6)=i16 0) -> (F-format string=w217:string)  [unwired: 2 in]
            n86 = Equal?(x=w229, y=w226) -> (x = y?=w222:bool)
            n87 = Equal?(x=w227, y=w226) -> (x = y?=w223:bool)
            n88 = case shown="False" w222 {
              tunnel: w225 -> [w240 w248]
              tunnel: [w240 w247] -> w224
              tunnel: w222 -> [_ w246]
              tunnel: w221 -> [_ w245]
              tunnel: w217 -> [_ w244]
              frame False {
              }
              frame True {
                n89 = Replace Array Subset(array=w245, new element=w244, index (row)=0, index (col)=1 ("disabled index (col)")) -> (w241:string[][])
                n90 = Bundle By Name(cluster=w248, "Dryer Out.Hist Record"=w241, "Restart Ready?"=w246) -> (w247:T6)
              }
            }
            n91 = case shown="True" w223 {
              tunnel: [_ "Increment Count" ("State(s) in Front (\"\")")] -> w228
              frame False {
              }
              frame True {
              }
            }
          }
          frame True {
            # "If status is the same,\ndon't do extra steps."
          }
        }
        n92 = call <vilib>:"Add State(s) to Queue__jki_lib_state_machine.vi"("State(s) in Front (\"\")"=w208, "State(s) in (\"\")"=w215) -> ("States Out"=w214:string)  [unwired: 13 in]
      }
      frame "Check for Index" {
        w257 = 3  # ASCII Location
        # "Your code here.\n(You can make a copy of, or modify, this frame)"
        n93 = Unbundle By Name(w259) -> ("Dryer Out.Sample Record"=w260:string[])
        n94 = Index Array(array=w260, index=w257) -> (element=w256:string)
        n95 = Match Pattern(string=w256, regular expression="Cycle Index: 00") -> (after substring=w252:string, offset past match=w254:i32)  [unwired: 1 in, 2 out]
        n96 = Greater Or Equal To 0?(x=w254) -> (x >= 0?=w253:bool)
        n97 = case shown="False" w253 {
          tunnel: w259 -> [w264 w270]
          tunnel: [w264 w269] -> w258
          tunnel: w252 -> [_ w268]
          frame False {
          }
          frame True {
            # "the read value is 1 off of the value expected by the techs."
            # "old stat"
            n98 = Scan From String(format string="%2s", input string=w268) -> (output 1=w266:string)  [unwired: 3 in, 3 out]
            n99 = case shown="\"06\"" w266 {
              tunnel: ["??" ("Dryer Out.Cycle Index") "01" ("Dryer Out.Cycle Index") "02" ("Dryer Out.Cycle Index") "03" ("Dryer Out.Cycle Index") "04" ("Dryer Out.Cycle Index") "05" ("Dryer Out.Cycle Index") "06" ("Dryer Out.Cycle Index") "07" ("Dryer Out.Cycle Index")] -> w265
              frame "False", Default {
              }
              frame "00" {
              }
              frame "01" {
              }
              frame "02" {
              }
              frame "03" {
              }
              frame "04" {
              }
              frame "05" {
              }
              frame "06" {
              }
            }
            n100 = Bundle By Name(cluster=w270, "Dryer Out.Cycle Index"=w265) -> (w269:T6)
          }
        }
        n101 = call <vilib>:"Add State(s) to Queue__jki_lib_state_machine.vi"("State(s) in (\"\")"=w263) -> ("States Out"=w262:string)  [unwired: 14 in]
      }
      frame "Update Time On" {
        w282 = dbl[] [400.0, 2000.0, 4000.0]  # Hours for Audit Alert
        # "if the cycle is running, increment the time with the amount of time elapsed from the last time. \nIf the time crossed one of the audit alert thresholds, set the audit alert indicators."
        n102 = Unbundle By Name(w288) -> ("Dryer Out.Audit Alert"=w279:bool, "Dryer Out.Sample Record"=w290:string[], "Dryer Status Serial Data In.Time(S)"=w289:dbl, "Dryer Out.Dryer Details.Time On Day"=w284:string, "Dryer Out.Dryer Details.Time On Night"=w283:string, "Dryer Status Serial Data In.Last Read Status"=w285:T4)
        n103 = Equal?(x=w285, y=Dryer_Status_Ctrl."Cycle Running" ("Status")) -> (x = y?=w291:bool)
        n104 = Multiply(x=w282, y=3600.0 ("Seconds Out")) -> (x*y=w280:dbl[])
        n105 = case shown="True" w291 {
          tunnel: w290 -> [w321 w341]
          tunnel: w289 -> [w319 w339]
          tunnel: w288 -> [w323 w343]
          tunnel: [w322 w342] -> w287
          tunnel: w284 -> [w314 _]
          tunnel: w283 -> [w312 _]
          tunnel: w280 -> [w303 _]
          tunnel: w279 -> [w299 _]
          frame True {
            # "increment>"
            # "cumulitive time>"
            # "set audit alert if threshold times crossed."
            # "Increment>"
            # "other shift  time>"
            # "Cum Time"
            # "Current Rec Time"
            # "Last Time"
            n106 = local read "Day Shift?"() -> (w310:bool)
            n107 = case shown="False" w310 {
              tunnel: w314 -> [w331 w336]
              tunnel: [w333 w336] -> w313
              tunnel: w312 -> [w333 w334]
              tunnel: [w332 w335] -> w304
              tunnel: [w331 w334] -> w305
              frame False {
                n108 = call "Type Conv Seconds - Time String.vi"("Time String In"=w331) -> ("Seconds Out"=w332:dbl)  [unwired: 9 in, 1 out]
              }
              frame True {
                n109 = call "Type Conv Seconds - Time String.vi"("Time String In"=w334) -> ("Seconds Out"=w335:dbl)  [unwired: 9 in, 1 out]
              }
            }
            n110 = Index Array(array=w321, index #1=0 ("index (row)")) -> (element #1=w326:string)  [unwired: 1 in, 1 out]
            n111 = Fract/Exp String To Number(string=w326) -> (number=w324:dbl)  [unwired: 3 in, 1 out]
            n112 = call "Type Conv Seconds - Time String.vi"("Time String In"=w313) -> ("Seconds Out"=w315:dbl)  [unwired: 9 in, 1 out]
            n113 = Subtract(x=w319, y=w324) -> (x-y=w296:dbl)
            n114 = Add(x=w296, y=w315) -> (x+y=w311:dbl)
            n115 = Add(x=w311, y=w304) -> (x+y=w297:dbl)
            n116 = Subtract(x=w297, y=w296) -> (x-y=w295:dbl)
            n117 = Number To Fractional String(number=w319) -> (F-format string=w318:string)  [unwired: 3 in]
            n118 = call "Type Conv Seconds - Time String.vi"("Seconds In"=w311) -> ("Time String Out"=w307:string)  [unwired: 9 in, 1 out]
            n119 = In Range and Coerce(upper limit=w297, x=w303, lower limit=w295) -> (In Range?=w302:bool[])  [unwired: 1 out]
            n120 = call "Type Conv Seconds - Time String.vi"("Seconds In"=w297) -> ("Time String Out"=w309:string)  [unwired: 9 in, 1 out]
            n121 = Or Array Elements(Boolean array=w302) -> (logical OR=w301:bool)
            n122 = Replace Array Subset(array=w321, new element #1=w309, index #1=2 ("index (row)"), new element #2=w318, index #2=0 ("index")) -> (w320:string[])
            n123 = Select(t=TRUE ("logical OR"), s=w301, f=w299) -> (s? t:f=w298:bool)
            n124 = case shown="False" w310 {
              tunnel: [w327 w330] -> w308
              tunnel: w307 -> [w328 w330]
              tunnel: [w328 w329] -> w306
              tunnel: w305 -> [w327 w329]
              frame False {
              }
              frame True {
              }
            }
            n125 = Bundle By Name(cluster=w323, "Dryer Out.Audit Alert"=w298, "Dryer Out.Sample Record"=w320, "Dryer Out.Dryer Details.Time On Day"=w308, "Dryer Out.Dryer Details.Time On Night"=w306, "Dryer Out.Dryer Details.Total Time On"=w309) -> (w322:T6)
          }
          frame False {
            # "Just update Record Time"
            n126 = Number To Fractional String(number=w339) -> (F-format string=w337:string)  [unwired: 3 in]
            n127 = Replace Array Subset(array=w341, new element=w337, index=0 ("index (row)")) -> (w340:string[])
            n128 = Bundle By Name(cluster=w343, "Dryer Out.Sample Record"=w340) -> (w342:T6)
          }
        }
        n129 = call <vilib>:"Add State(s) to Queue__jki_lib_state_machine.vi"("State(s) in (\"\")"=w294) -> ("States Out"=w293:string)  [unwired: 14 in]
      }
      frame "Update Com Info" {
        # "Put Dryer Serial Data in into dryer out sample record."
        # "Your code here.\n(You can make a copy of, or modify, this frame)"
        n130 = Unbundle By Name(w360) -> ("Temperature Fault"=w346:bool, "Dryer Out.Sample Record"=w358:string[], "Dryer Status Serial Data In"=w357:T3)
        n131 = Unbundle By Name(w357) -> ("Err Count"=w353:u32, "Color"=w347:u32, "Last Read Status"=w354:T4, "Command:Data"=w349:string)
        n132 = global read "Globals Wilt.vi" "Temperature Fault"() -> (w345:u32)
        n133 = disable-structure shown="Enabled" {
          disable-tunnel: w349 -> [w369 w370]
          disable-tunnel: [w364 w370] -> w348
          frame Enabled {
            w365 = " :: " ("replace string (\"\")")
            n134 = Search and Replace String(input string=w369, search string="\r\n", replace string=w365) -> (result string=w367:string)  [unwired: 5 in, 3 out]
            n135 = Search and Replace String(input string=w367, search string="\r", replace string=w365) -> (result string=w364:string)  [unwired: 5 in, 3 out]
          }
          frame Disabled {
          }
        }
        n136 = Select(t=w345, s=w346, f=w347) -> (s? t:f=w344:u32)
        n137 = call "Type Conv - Dryer Status to Txt.vi"("Status"=w354) -> ("Ring Text.Text"=w356:string)  [unwired: 10 in]
        n138 = To Long Integer(number=w353) -> (32bit integer=w352:i32)
        n139 = Replace Array Subset(array=w358, new element #1=w348, index #1=3 ("disabled index (col)"), new element #2=w356, index #2=4 ("disabled index (col)")) -> (w355:string[])
        n140 = Bundle By Name(cluster=w360, "Dryer Out.Bad Com Count"=w352, "Dryer Out.Status Color"=w344, "Dryer Out.Sample Record"=w355) -> (w359:T6)
        n141 = call <vilib>:"Add State(s) to Queue__jki_lib_state_machine.vi"("State(s) in (\"\")"=w363) -> ("States Out"=w362:string)  [unwired: 14 in]
      }
      frame "Update Views from Sample" {
        w371 = 4  # Tmax
        w372 = 3  # L2max
        w373 = 2  # L1max
        w374 = 0  # CC
        w377 = 7  # Trmb(col)
        w378 = 4  # Tmax
        w395 = 6  # L2 (col)
        w396 = 5  # L1 (col)
        w399 = 3  # L2max
        w400 = 2  # L1max
        w401 = 1  # t-comp
        w403 = 0 ("index (row)")
        w402 = 0  # CC
        w406 = 2  # Cum. Time(col)
        w407 = 3  # ASCII(col)
        w408 = 4  # Status (col)
        w409 = 1  # CC(col)
        # "Updates the view data, and the History data."
        # "Using Sample Record:  Update Dryer Out Record and compare to previous Hist Record to see if max's are exceeded."
        n142 = Unbundle By Name(w414) -> ("Dryer Out.Sample Record"=w412:string[], "Dryer Out.Hist Record"=w405:string[][])
        n143 = Index Array(array=w405, index (row) #1=w374, index (col) #1=w373, index (row) #2=w374, index (col) #2=w372, index (row) #3=w374, index (col) #3=w371) -> (element #1=w389:string, element #2=w388:string, element #3=w375:string)
        n144 = Index Array(array=w412, index #1=w409, index #2=w408, index #3=w407, index #4=w406, index #5=w396, index #6=w395, index #7=w377) -> (element #1=w398:string, element #2=w411:string, element #3=w410:string, element #4=w397:string, element #5=w390:string, element #6=w387:string, element #7=w376:string)
        n145 = Fract/Exp String To Number(string=w390) -> (number=w392:dbl)  [unwired: 3 in, 1 out]
        n146 = Fract/Exp String To Number(string=w389) -> (number=w391:dbl)  [unwired: 3 in, 1 out]
        n147 = Fract/Exp String To Number(string=w387) -> (number=w393:dbl)  [unwired: 3 in, 1 out]
        n148 = Fract/Exp String To Number(string=w388) -> (number=w394:dbl)  [unwired: 3 in, 1 out]
        n149 = Fract/Exp String To Number(string=w376) -> (number=w381:dbl)  [unwired: 3 in, 1 out]
        n150 = Fract/Exp String To Number(string=w375) -> (number=w380:dbl)  [unwired: 3 in, 1 out]
        n151 = Max & Min(x=w392, y=w391) -> (max(x,y)=w383:dbl)  [unwired: 1 out]
        n152 = Max & Min(x=w393, y=w394) -> (max(x,y)=w384:dbl)  [unwired: 1 out]
        n153 = Max & Min(x=w381, y=w380) -> (max(x,y)=w382:dbl)  [unwired: 1 out]
        n154 = Number To Fractional String(number=w383) -> (F-format string=w386:string)  [unwired: 3 in]
        n155 = Number To Fractional String(number=w384) -> (F-format string=w385:string)  [unwired: 3 in]
        n156 = Number To Fractional String(number=w382) -> (F-format string=w379:string)  [unwired: 3 in]
        n157 = Replace Array Subset(array=w405, new element #1=w398, index (row) #1=w403, index (col) #1=w402, new element #2=w397, index (row) #2=w403, index (col) #2=w401, new element #3=w386, index (row) #3=w403, index (col) #3=w400, new element #4=w385, index (row) #4=w403, index (col) #4=w399, new element #5=w379, index (row) #5=w403, index (col) #5=w378) -> (w404:string[][])
        n158 = Bundle By Name(cluster=w414, "Dryer Out.Dryer Details.Status"=w411, "Dryer Out.Dryer Details.Debug ASCII"=w410, "Dryer Out.Dryer Details.Total Time On"=w397, "Dryer Out.Hist Record"=w404) -> (w413:T6)
        n159 = call <vilib>:"Add State(s) to Queue__jki_lib_state_machine.vi"("State(s) in (\"\")"=w417) -> ("States Out"=w416:string)  [unwired: 14 in]
      }
      frame "-----If Status Has Changed-----" {
        # "Template Separator\n(You can make a copy of, or modify, this frame)"
        n160 = call <vilib>:"Add State(s) to Queue__jki_lib_state_machine.vi"("State(s) in (\"\")"=w421) -> ("States Out"=w420:string)  [unwired: 14 in]
      }
      frame "Update History Data" {
        w425 = 10  # Max Record Size
        w431 = "0" ("element")
        # "This may be the memory leak.  Limit the number of  historical records to max record size."
        # "Insert new record on top of stack.  This will be updated as time goes on during the cycle.  This happens when there is an increment count."
        n161 = Unbundle By Name(w437) -> ("Dryer Out.Hist Record"=w423:string[][], "Dryer Out.Day Cycle Count"=w432:i32)
        n162 = Array Size(array=w423) -> (size(s)=w429:i32[])
        n163 = Index Array(array=w429, index=0) -> (element=w426:i32)
        n164 = Number To Fractional String(number=w432) -> (F-format string=w435:string)  [unwired: 3 in]
        n165 = Greater?(x=w426, y=w425) -> (0:w427:bool)
        n166 = Subtract(x=w426, y=w425) -> (x-y=w424:i32)
        n167 = Build Array(w435, w431, w431, w431, w431) -> (w434:string[])
        n168 = case shown="False" w427 {
          tunnel: w423 -> [w441 w444]
          tunnel: w424 -> [_ w443]
          tunnel: [w441 w442] -> w422
          frame False {
          }
          frame True {
            n169 = Delete From Array(array=w444, length=w443) -> (array with subset deleted=w442:string[][])  [unwired: 2 in, 1 out]
          }
        }
        n170 = Build Array (concatenate)(w434, w422) -> (w433:string[][])
        n171 = call "E-Time.vi"() -> ("Elapsed Time (sec)"=w430:dbl)  [unwired: 9 in, 2 out]
        n172 = Bundle By Name(cluster=w437, "Dryer Out.Hist Record"=w433, "Dryer Out.Current Run Start Time"=w430) -> (w436:T6)
        n173 = call <vilib>:"Add State(s) to Queue__jki_lib_state_machine.vi"("State(s) in (\"\")"=w440) -> ("States Out"=w439:string)  [unwired: 14 in]
      }
      frame "Increment Count" {
        w455 = 1  # Cycle Count (col)
        # "Adds one to count in the sample record, and calls update history data (which creates a new history record)."
        n174 = Unbundle By Name(w460) -> ("Dryer Out.Sample Record"=w461:string[], "Dryer Out.Dryer Details.Cycle Count Day"=w454:string, "Dryer Out.Dryer Details.Cycle Count Night"=w453:string, "Day Shift?"=w445:bool)
        n175 = Decimal String To Number(string=w454) -> (number=w452:i32)  [unwired: 2 in, 1 out]
        n176 = Decimal String To Number(string=w453) -> (number=w451:i32)  [unwired: 2 in, 1 out]
        n177 = case shown="True" w445 {
          tunnel: w452 -> [w465 w470]
          tunnel: w451 -> [w467 w468]
          tunnel: [w465 w469] -> w447
          tunnel: [w466 w468] -> w446
          frame False {
            n178 = Increment(x=w467) -> (x+1=w466:i32)
          }
          frame True {
            n179 = Increment(x=w470) -> (x+1=w469:i32)
          }
        }
        n180 = Add(x=w447, y=w446) -> (x+y=w450:i32)
        n181 = Number To Decimal String(number=w450) -> (decimal integer string=w457:string)  [unwired: 1 in]
        n182 = Replace Array Subset(array=w461, new element=w457, index=w455) -> (w458:string[])
        n183 = Number To Decimal String(number=w447) -> (decimal integer string=w449:string)  [unwired: 1 in]
        n184 = Number To Decimal String(number=w446) -> (decimal integer string=w448:string)  [unwired: 1 in]
        n185 = Bundle By Name(cluster=w460, "Dryer Out.Sample Record"=w458, "Dryer Out.Dryer Details.Cycle Count Day"=w449, "Dryer Out.Dryer Details.Cycle Count Night"=w448, "Dryer Out.Day Cycle Count"=w447, "Dryer Out.Night Cycle Count"=w446) -> (w459:T6)
        n186 = call <vilib>:"Add State(s) to Queue__jki_lib_state_machine.vi"("State(s) in Front (\"\")"="Update History Data" ("State(s) in Front (\"\")"), "State(s) in (\"\")"=w464) -> ("States Out"=w463:string)  [unwired: 13 in]
      }
    }
  }
  n187 = Unbundle By Name(w2) -> ("Restart Ready?"=→"Restart Ready?":bool)
